vi "Progress Bar Settings.vi"(4 "Seconds Before Showing (1)":dbl=1.0, 6 "Show on Taskbar (Win7 Only) (f)":bool, 7 "Show Time (f)":bool, 10 "Window Title (Progress)":string="Progress", 11 "Show Abort (f)":bool) -> (3 "MGI_Progress Bar Settings":refnum<class "Progress Bar Settings.lvclass">)   [LabVIEW 2020, in "Progress Bar Settings.lvclass"]
doc: "Constructor\n\nCopyright: MGI\nAuthored by: Derek Trepanier"
uses:
  <userlib>/_MGI/User Interface/Progress Bar/Progress Bar Settings/Progress Bar Settings.lvclass
  <userlib>/_MGI/User Interface/Progress Bar/Progress Bar Settings/Progress Bar Settings.lvclass/Progress Bar Settings.ctl
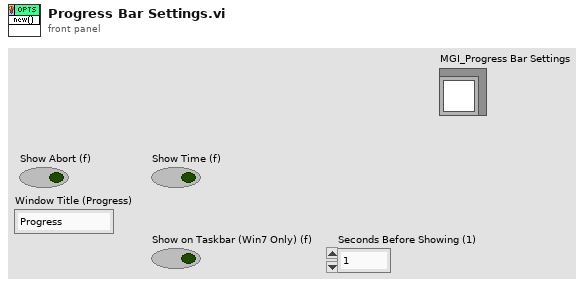
[diagram p1: front panel]
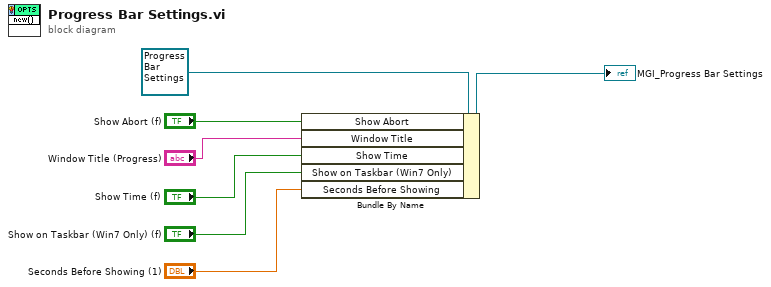
[diagram p0: block diagram]
diagram:
  n1 = Bundle By Name(cluster=refnum<class "Progress Bar Settings.lvclass"> refnum ("Prog Bar Settings in"), "Show Abort"="Show Abort (f)", "Window Title"="Window Title (Progress)", "Show Time"="Show Time (f)", "Show on Taskbar (Win7 Only)"="Show on Taskbar (Win7 Only) (f)", "Seconds Before Showing"="Seconds Before Showing (1)") -> (→"MGI_Progress Bar Settings":refnum<class "Progress Bar Settings.lvclass">)
